vi "Czytanie.vi"() -> ()   [LabVIEW 2020]
uses:
  <vilib>/userdefined/High Color/IMAQdx.ctl
  <vilib>/vision/driver/NI_Vision_Acquisition_Software.lvlib
  <vilib>/vision/NI_Vision_Development_Module.lvlib
panel:
  out "Plate Number":string
  in  "Rectangle":T1 {"Rotation" min=-90.0 max=90.0 step=1.0 format="%.2f"; "Left" scale=0.0..1024.0; "Right" scale=0.0..1024.0}
  in  "File Path":path
  out "Plate":T2(plugin-control)
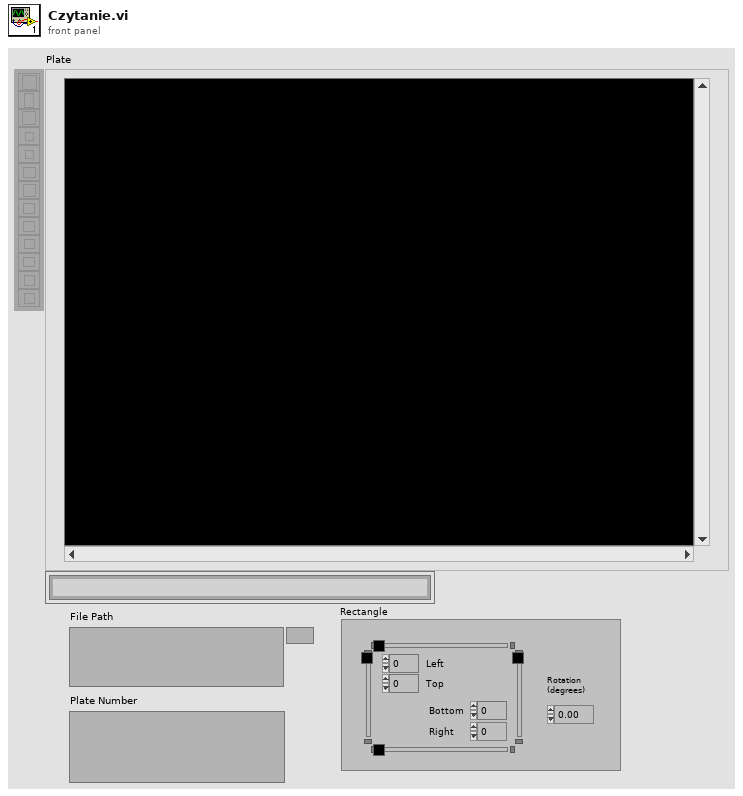
[diagram p1: front panel]
types:
  T1 = typedef "IMAQ Rectangle" = cluster{"Left":i32, "Top":i32, "Right":i32, "Bottom":i32, "Rotation":dbl}
  T2 = typedef "IMAQ Image.ctl" = refnum<image>
  T3 = typedef "IMAQdx.ctl" = refnum<k21>
  T4 = typedef "IMAQ OCR Session.ctl" = refnum<k1>
  T5 = typedef "ROI Descriptor" = cluster{"Global Rectangle":i32[], "Contours":cluster{"ID":enum32{"External", "Internal"}, "Type":u32, "Coordinates":i32[]}[]}
  T6 = cluster{"Global Rectangle":i32[], "Contours":cluster{"ID":enum32{"External", "Internal"}, "Type":u32, "Coordinates":i32[]}[]}
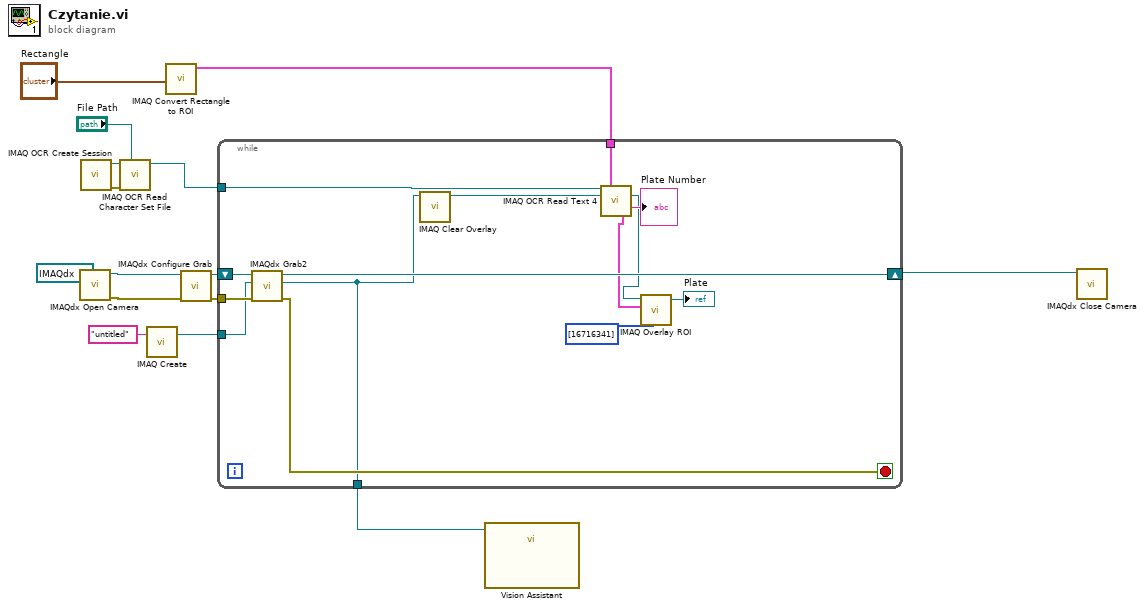
[diagram p0: block diagram]
diagram:
  n1 = call <vilib>:"IMAQdx Open Camera.vi"("Session In"=T3 "cam0") -> ("error out"=w11:errorcluster, "Session Out"=w12:T3)  [unwired: 9 in]
  n2 = call "IMAQ OCR Create Session"() -> ("error out"=w7:errorcluster, "IMAQ OCR Session"=w6:T4)  [unwired: 10 in]
  n3 = call "IMAQ OCR Read Character Set File"("File Path"="File Path", "error in (no error)"=w7, "IMAQ OCR Session"=w6) -> ("IMAQ OCR Session (dup)"=w4:T4)  [unwired: 6 in, 2 out]
  n4 = call "IMAQ Create"("Image Name"="untitled") -> ("New Image"=w10:T2)  [unwired: 4 in, 1 out]
  n5 = call "IMAQ Convert Rectangle to ROI"("Rectangle"="Rectangle") -> ("ROI Descriptor"=w2:T5)  [unwired: 8 in, 1 out]
  n6 = call <vilib>:"IMAQdx Configure Grab.vi"("error in"=w11, "Session In"=w12) -> ("error out"=w14:errorcluster, "Session Out"=w13:T3)  [unwired: 8 in]
  n7 = while {
    tunnel: w14 -> [w29]
    tunnel: w10 -> [w27]
    shift-right: [w26] -> w9
    shift-left: w13 -> [w28]
    tunnel: w4 -> [w25]
    tunnel: w2 -> [w24]
    tunnel: [w16] -> w1
    stop <- w18 stop-if-true
    n8 = call <vilib>:"IMAQdx Grab2.vi"("error in"=w29, "Image In"=w27, "Session In"=w28) -> ("error out"=w18:errorcluster, "Image Out"=w16:T2, "Session Out"=w26:T3)  [unwired: 5 in, 1 out]
    n9 = call "IMAQ Clear Overlay"("Image"=w16) -> ("Image Out"=w17:T2)  [unwired: 9 in, 1 out]
    n10 = call "IMAQ OCR Read Text 4"("IMAQ OCR Session"=w25, "ROI Descriptor"=w24, "Image"=w17) -> ("Image (dup)"=w21:T2, "Read String"=→"Plate Number":string, "ROI Bounding Characters"=w20:T6)  [unwired: 6 in, 4 out]
    n11 = call "IMAQ Overlay ROI"("Colors (Green)"=u32[] [16716341], "ROI Descriptor"=w20, "Image"=w21) -> ("Image Out"=→"Plate":T2)  [unwired: 7 in, 1 out]
  }
  n12 = call "Vision Assistant"("Image In"=w1) -> ()  [unwired: 25 in, 2 out]
  n13 = call <vilib>:"IMAQdx Close Camera.vi"("Session In"=w9) -> ()  [unwired: 10 in, 1 out]
